vi "move_x.vi"(5 "^":bool, 6 "step size":dbl, 7 "v":bool, 8 "error in (no error)":errorcluster, 9 "x":dbl, 10 "handle in":i32, 11 "keys pressed":T1(array[ring])) -> (0 "error out":errorcluster, 3 "handle out":i32)   [LabVIEW 2019]
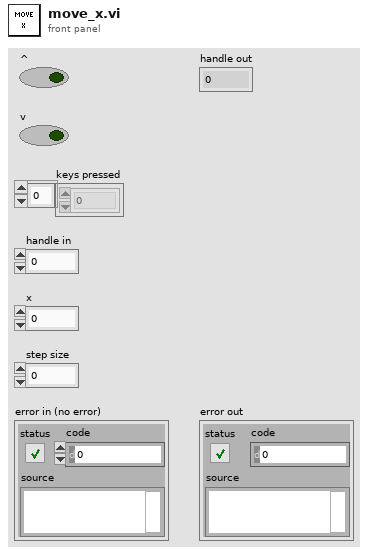
[diagram p1: front panel]
types:
  T1 = enum16{"0", "1", "2", "3", "4", "5", "6", "7", "8", "9", "A", "B", "C", "D", "E", "F", "G", "H", "I", "J", "K", "L", "M", "N", "O", "P", "Q", "R", "S", "T", "U", "V", "W", "X", "Y", "Z", "F1", "F2", "F3", "F4", "F5", "F6", "F7", "F8", "F9", "F10", "F11", "F12", "F13", "F14", "F15", "ADD", "BACK", "BACKSLASH", "CAPITAL", "COMMA", "DECIMAL", "DELETE", "DIVIDE", "DOWN", "END", "EQUALS", "ESCAPE", "GRAVE (`)", "HOME", "INSERT", "LBRACKET", "LCONTROL", "LEFT", "L ALT", "LSHIFT", "LWIN", "MINUS", "MULTIPLY", "NEXT", "NUMLOCK", "NUMPAD_0", "NUMPAD_1", "NUMPAD_2", "NUMPAD_3", "NUMPAD_4", "NUMPAD_5", "NUMPAD_6", "NUMPAD_7", "NUMPAD_8", "NUMPAD_9", "PAUSE", "PERIOD", "PRIOR (PG UP)", "RBRACKET", "RCONTROL", "RETURN", "RIGHT", "R ALT", "RSHIFT", "RWIN", "SCROLL", "SEMICOLON", "SLASH", "SPACE", "SUBTRACT", "TAB", "UP", "ENTER (num pad)", "' (quote)"}[]
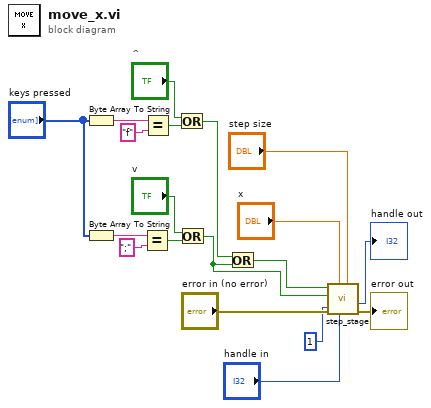
[diagram p0: block diagram]
diagram:
  n1 = Byte Array To String(unsigned byte array="keys pressed") -> (string=w9:string)
  n2 = Byte Array To String(unsigned byte array="keys pressed") -> (string=w8:string)
  n3 = Equal?(x=w8, y=";") -> (x = y?=w6:bool)
  n4 = Equal?(x=w9, y="f") -> (x = y?=w7:bool)
  n5 = Or(x="^", y=w7) -> (x .or. y?=w5:bool)
  n6 = Or(x="v", y=w6) -> (x .or. y?=w2:bool)
  n7 = Or(x=w5, y=w2) -> (x .or. y?=w1:bool)
  n8 = call "step_stage.vi"("axis"=u32 1, "step"="step size", "handle"="handle in", "position"="x", "error in"="error in (no error)", "+/-"=w2, "move"=w1) -> ("error out"=→"error out":errorcluster, "handle out"=→"handle out":i32)  [unwired: 3 in]
